vi "convert to HEX string.vi"(11 "String In(binary)":string) -> (3 "String Out (hexa)":string)   [LabVIEW 2018]
panel:
  in  "error in (no error)":errorcluster
  out "error out":errorcluster
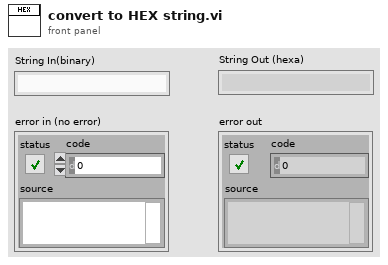
[diagram p1: front panel]
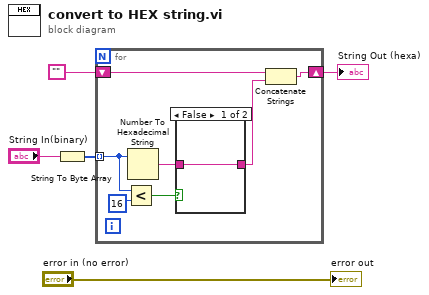
[diagram p0: block diagram]
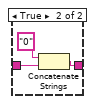
[diagram p2: hidden frame]
diagram:
  n1 = String To Byte Array(string="String In(binary)") -> (unsigned byte array=w5:u8[])
  n2 = for {
    tunnel: w5 -> [w11] mode=indexing
    shift-right: [w8] -> w2
    shift-left: "" -> [w7]
    n3 = Less?(x=w11, y=u8 16) -> (x < y?=w10:bool)
    n4 = Number To Hexadecimal String(2:w11) -> (0:w9:string)  [unwired: 1 in]
    n5 = case shown="False" w10 {
      tunnel: w9 -> [w13 w16]
      tunnel: [w13 w14] -> w6
      frame False {
      }
      frame True {
        n6 = Concatenate Strings("0", w16) -> (w14:string)
      }
    }
    n7 = Concatenate Strings(w7, w6) -> (w8:string)
  }
  "String Out (hexa)" <- w2
  "error out" <- "error in (no error)"
